vi "MQTT Chat Launcher.vi"() -> ()   [LabVIEW 2020, in "MQTT Chat.lvlib"]
uses:
  MQTT Chat.lvlib
  Simple Chat/Simple Chat/Simple Chat.lvclass
  C:/Program Files/National Instruments/LabVIEW 2020/vi.lib/ActorFramework/Actor/Actor.lvclass
  <vilib>/LabVIEW Open Source Project/MQTT Client/Client class/Client.lvclass/Client.ctl
  <vilib>/G Open Source Project for LabVIEW/MQTT Broker/Server class/Server.lvclass/Server.ctl
  <vilib>/LabVIEW Open Source Project/MQTT Control Packets/Control Packets/ControlPacket/ControlPacket.lvclass/ControlPacket.ctl
  <vilib>/ActorFramework/Message Enqueuer/Message Enqueuer.lvclass/Message Enqueuer.ctl
  <vilib>/ActorFramework/Message Enqueuer/Enqueue.vi
  <vilib>/LabVIEW Open Source Project/MQTT TCP Connection/MQTT_TCP/Connection/TCPConnection.lvclass
  C:/Program Files/National Instruments/LabVIEW 2020/vi.lib/LabVIEW Open Source Project/Connection/Connection/Connection.lvclass
  C:/Program Files/National Instruments/LabVIEW 2020/vi.lib/LabVIEW Open Source Project/MQTT Connection/MQTT_Connection/Connection/Connection.lvclass
  <vilib>/LabVIEW Open Source Project/MQTT Client/Client class/Client.lvclass
  C:/Program Files/National Instruments/LabVIEW 2020/vi.lib/LabVIEW Open Source Project/MQTT Connection/MQTT_Base/Base Class/MQTT_Base.lvclass
  <vilib>/G Open Source Project for LabVIEW/MQTT Broker/Server class/Server.lvclass
  AF MQTT Channel/AF MQTT Message Channel/AF MQTT Message Channel.lvclass
  E:/Labview/LV 2020/Libs/Actor Pub Sub/Source/Actor Pub Sub Channels/Pub Sub Message Channel/Pub Sub Message Channel.lvclass
  <vilib>/LabVIEW Open Source Project/MQTT Control Packets/Control Packets/PUBLISH/PUBLISH.lvclass
  C:/Program Files/National Instruments/LabVIEW 2020/vi.lib/LabVIEW Open Source Project/MQTT Control Packets/Control Packets/ControlPacket/ControlPacket.lvclass
  <vilib>/ActorFramework/Stop Msg/Stop Msg.lvclass
  C:/Program Files/National Instruments/LabVIEW 2020/vi.lib/ActorFramework/Message/Message.lvclass
  Actor Pub Sub Channels/Helpers/Get Topic Enqueuer.vi
  <vilib>/ActorFramework/Message Priority Queue/Priority Enqueue.vi
  <vilib>/LabVIEW Open Source Project/MQTT Connection/MQTT_Base/Base Class/MQTT_Base.lvclass
  Actor Pub Sub Channels/Actor Pub Sub Channels.lvlib
  E:/Labview/LV 2020/Libs/Actor Pub Sub/Source/AF MQTT Channel/AF MQTT Message Channel/AF MQTT Message Channel.lvclass
  <vilib>/LabVIEW Open Source Project/MQTT Control Packets/Control Packets/ControlPacket/ControlPacket.lvclass
  <vilib>/ActorFramework/Actor/Actor.lvclass
  E:/Labview/LV 2020/Libs/Actor Pub Sub/Source/Examples/Simple Chat/Simple Chat/Simple Chat.lvclass
  E:/Labview/LV 2020/Libs/Actor Pub Sub/Source/Actor Pub Sub Channels/PubSub Status Reciever Interface/PubSub Status Receiver Interface.lvclass
  E:/Labview/LV 2020/Libs/Actor Pub Sub/Source/Examples/Simple Chat/Message Reciever Interface/Message Receiver Interface.lvclass
panel:
  out "String":string
  in  "stop":bool
  in  "Start Chat":bool
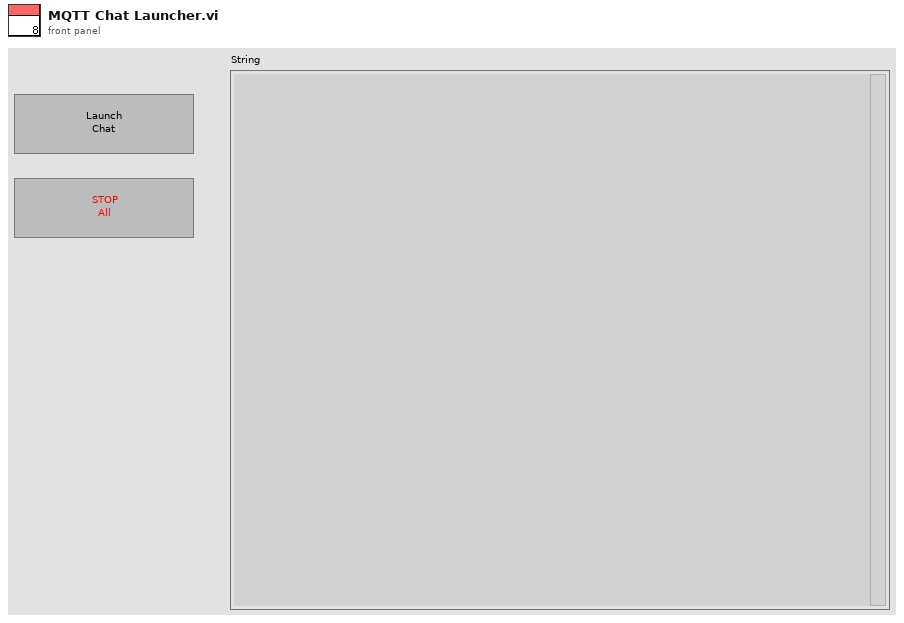
[diagram p1: front panel]
types:
  T1 = typedef "MQTT Server.lvlib/Server.lvclass/Public Events -- cluster.ctl" = cluster{"NbConnections":refnum<user-event>, "Client Event":refnum<user-event>}
  T2 = typedef "MQTT Client.lvlib/Client.lvclass/Public Events -- cluster.ctl" = cluster{"Connection Status":refnum<user-event>, "Connected":refnum<user-event>, "Application Message":refnum<user-event>}
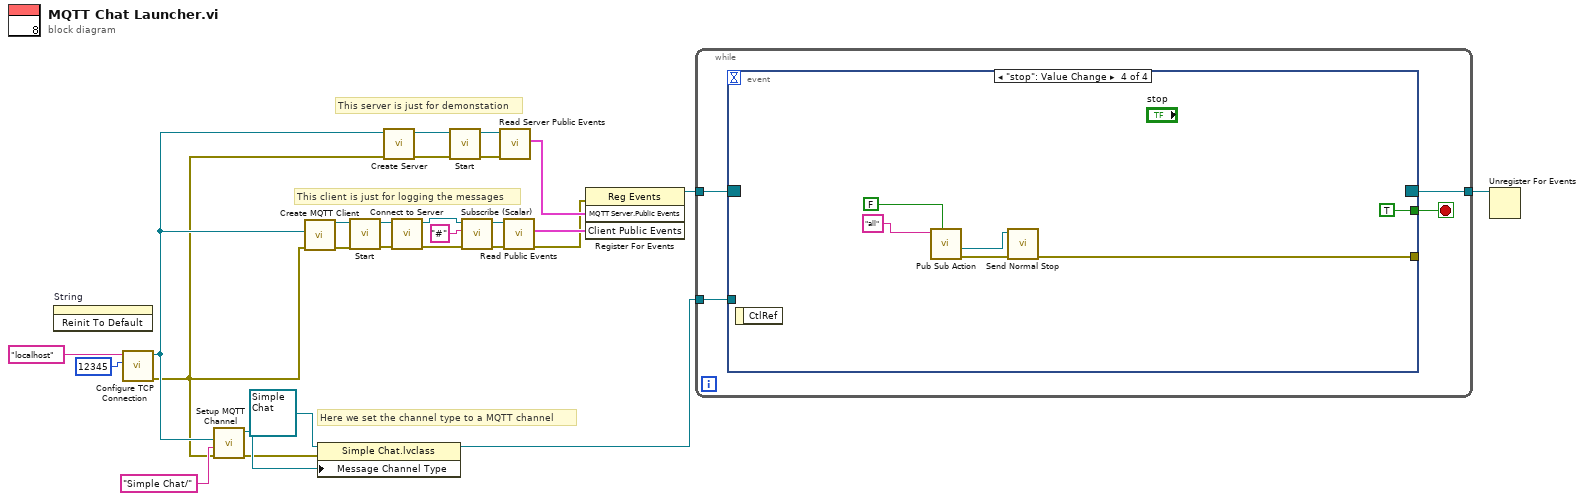
[diagram p0: block diagram]
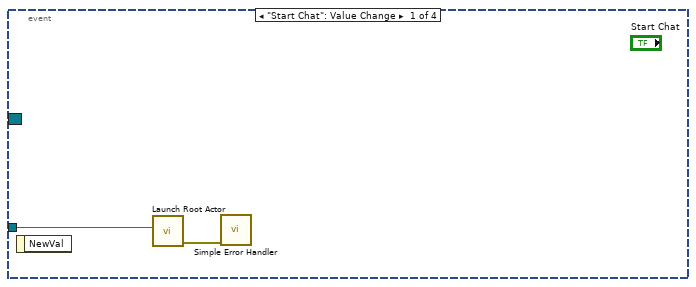
[diagram p2: hidden frame]
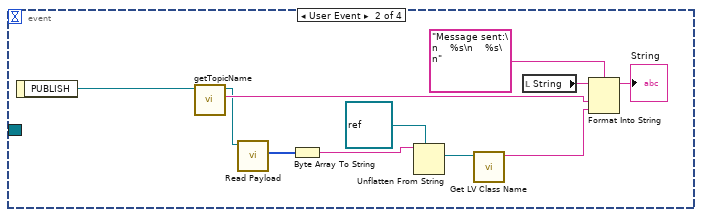
[diagram p3: hidden frame]
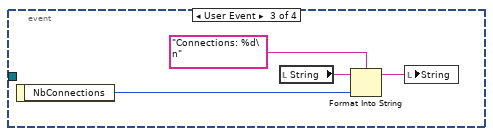
[diagram p4: hidden frame]
diagram:
  # "Here we set the channel type to a MQTT channel"
  # "This server is just for demonstation"
  # "This client is just for logging the messages"
  n1 = invoke on="String" class="Str" method="Reinit To Default"() -> ()  [unwired: 3 in, 3 out]
  n2 = call <vilib>:"Configure TCP Connection.vi"("remote port (80)"=u16 12345, "address (localhost)"="localhost") -> ("error out"=w1:errorcluster, "TCPConnection"=w13:refnum<class "TCPConnection.lvclass">)  [unwired: 8 in]
  n3 = call "Setup MQTT Channel.vi"("error in (no error)"=w1, "Topic Prefix"="Simple Chat/", "Connection Configuration"=w13) -> ("error out"=w20:errorcluster, "AF MQTT Message Channel out"=w21:refnum<class "AF MQTT Message Channel.lvclass">)  [unwired: 7 in]
  n4 = call <vilib>:"Create MQTT Client.vi"("error in (no error)"=w1, "Connection Configuration"=w13) -> ("error out"=w3:errorcluster, "Client out"=w12:refnum<class "Client.lvclass">)  [unwired: 8 in]
  n5 = property class="Simple Chat.lvclass"(reference=refnum<class "Simple Chat.lvclass"> refnum ("Simple Chat.lvlib:Simple Chat.lvclass"), error in=w20, "Message Channel Type"=w21) -> (reference out=w22:refnum<class "Simple Chat.lvclass">)  [unwired: 1 out]
  n6 = call <vilib>:"Start.vi"("error in (no error)"=w3, "MQTT_Base in"=w12) -> ("error out"=w10:errorcluster, "MQTT_Base out"=w11:refnum<class "Client.lvclass">)  [unwired: 7 in, 1 out]
  n7 = call <vilib>:"Create Server.vi"("error in (no error)"=w1, "Connection Configuration"=w13) -> ("error out"=w24:errorcluster, "Server"=w25:refnum<class "Server.lvclass">)  [unwired: 8 in]
  n8 = call <vilib>:"Connect to Server.vi"("error in (no error)"=w10, "Client in"=w11) -> ("error out"=w8:errorcluster, "Client out"=w9:refnum<class "Client.lvclass">)  [unwired: 6 in, 2 out]
  n9 = call <vilib>:"Start.vi"("error in (no error)"=w24, "MQTT_Base in"=w25) -> ("error out"=w18:errorcluster, "MQTT_Base out"=w19:refnum<class "Server.lvclass">)  [unwired: 7 in, 1 out]
  n10 = call <vilib>:"Subscribe (Scalar).vi"("error in (no error)"=w8, "Topic Filter"="#", "Client in"=w9) -> ("error out"=w5:errorcluster, "Client out"=w6:refnum<class "Client.lvclass">)  [unwired: 6 in, 1 out]
  n11 = call <vilib>:"Read Server Public Events.vi"("error in (no error)"=w18, "Server in"=w19) -> ("MQTT Server.Public Events"=w15:T1)  [unwired: 7 in, 2 out]
  n12 = call <vilib>:"Read Public Events.vi"("error in (no error)"=w5, "Client in"=w6) -> ("error out"=w2:errorcluster, "Client Public Events"=w4:T2)  [unwired: 7 in, 1 out]
  n13 = register-events(error in=w2, w15, w4) -> (reference out=w17:refnum<event-registration>)  [unwired: 1 in, 1 out]
  n14 = while {
    tunnel: w22 -> [w31]
    tunnel: w17 -> [w30]
    tunnel: [w29] -> w16
    stop <- w28 stop-if-true
    n15 = event shown="[3] \"stop\": Value Change" {
      selector: w30 -> [_ _ _ _]
      dyn-events: [_ _ _ _] -> w29
      timeout: _ -> [_ _ _ _]
      tunnel: w31 -> [w33 _ _ _]
      tunnel: [_ _ _ TRUE] -> w28
      tunnel: [_ _ _ w49] -> _
      event "Start Chat": Value Change {
        n16 = event-data() -> ()  [unwired: 1 in, 1 out]
        n17 = call <vilib>:"Launch Root Actor.vi"("Actor"=w33) -> ("error out"=w32:errorcluster)  [unwired: 9 in, 1 out]
        n18 = call <vilib>:"Simple Error Handler.vi"("error in (no error)"=w32) -> ()  [unwired: 4 in, 5 out]
      }
      event User Event {
        n19 = event-data() -> ("PUBLISH"=w44:refnum<class "PUBLISH.lvclass">)  [unwired: 1 in]
        n20 = call <vilib>:"getTopicName.vi"("PUBLISH in"=w44) -> ("Topic"=w41:string, "PUBLISH out"=w39:refnum<class "PUBLISH.lvclass">)  [unwired: 8 in, 1 out]
        n21 = call <vilib>:"Read Payload.vi"("ControlPacket in"=w39) -> ("Payload"=w38:u8[])  [unwired: 9 in, 1 out]
        n22 = Byte Array To String(unsigned byte array=w38) -> (string=w37:string)
        n23 = Unflatten From String(type=refnum<class> refnum ("LabVIEW Object"), binary string=w37) -> (value=w35:refnum<class>)  [unwired: 3 in, 2 out]
        n24 = call <vilib>:"Get LV Class Name.vi"("object"=w35) -> ("class name"=w34:string)  [unwired: 9 in, 1 out]
        n25 = local read "String"() -> (w43:string)
        n26 = Format Into String(format string="Message sent:\n    %s\n    %s\n", initial string=w43, w41, w34) -> (resulting string=→"String":string)  [unwired: 1 in, 1 out]
      }
      event User Event {
        n27 = event-data() -> ("NbConnections"=w46:u32)  [unwired: 1 in]
        n28 = local read "String"() -> (w48:string)
        n29 = Format Into String(format string="Connections: %d\n", initial string=w48, w46) -> (resulting string=w45:string)  [unwired: 1 in, 1 out]
        n30 = local write "String"(w45) -> ()
      }
      event "stop": Value Change {
        n31 = event-data() -> ()  [unwired: 1 in, 1 out]
        n32 = call-poly "Pub Sub Action.vi"("Create if not exist? (T)"=FALSE, "Topic"="all") -> ("error out"=w52:errorcluster, "Topic Enqueuer"=w53:refnum<class "Message Enqueuer.lvclass">)  [unwired: 6 in, 2 out]
        n33 = call <vilib>:"Send Normal Stop.vi"("error in (no error)"=w52, "Message Enqueuer"=w53) -> ("error out"=w49:errorcluster)  [unwired: 9 in]
      }
    }
  }
  n34 = Unregister For Events(event registration refnum=w16) -> ()  [unwired: 1 in, 1 out]
